vi "GEA2 Message to LEUI_LED with Binary conversion.vi"(5 "Ignore Brightness":bool, 7 "Raw Data In":string) -> (4 "Cycle Number":u32, 8 "LEUI_LEDs":T1)   [LabVIEW 2016, in "TLMB.lvlib"]
uses:
  Projects/TLMB.lvlib
  controls/LEUI_LEDs.ctl
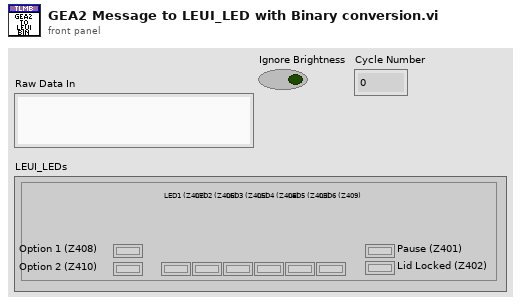
[diagram p1: front panel]
types:
  T1 = typedef "TLMB.lvlib/LEUI_LEDs.ctl" = cluster{"Pause (Z401)":bool, "Lid Locked (Z402)":bool, "LED1 (Z407)":bool, "LED2 (Z406)":bool, "LED3 (Z405)":bool, "LED4 (Z404)":bool, "LED5 (Z403)":bool, "LED6 (Z409)":bool, "Option 1 (Z408)":bool, "Option 2 (Z410)":bool}
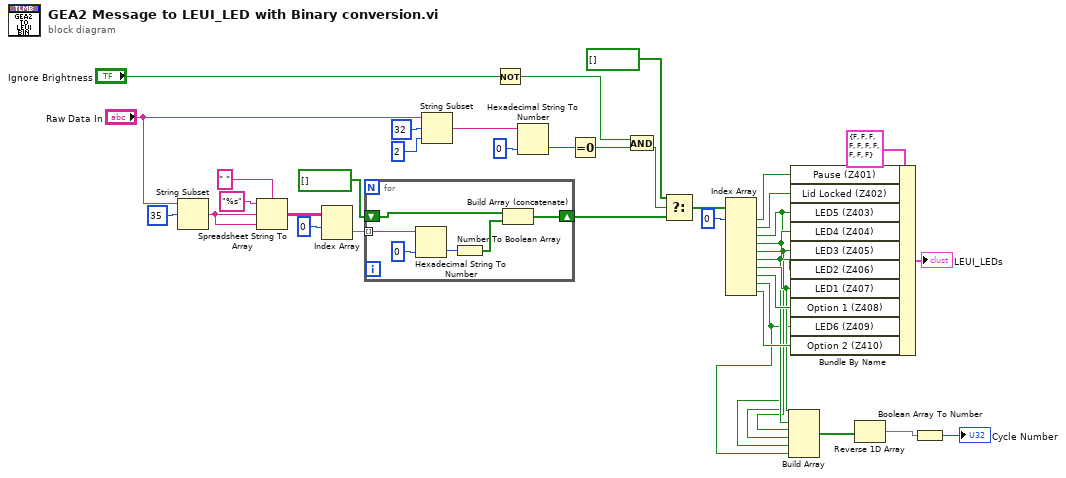
[diagram p0: block diagram]
diagram:
  n1 = String Subset(string="Raw Data In", offset (0)=35) -> (substring=w30:string)  [unwired: 1 in]
  n2 = Spreadsheet String To Array(delimiter (Tab)=" ", format string="%s", spreadsheet string=w30, array type (2D Dbl)=w30) -> (array=w34:string[][])
  n3 = Index Array(array=w34, index (row)=0) -> (element=w31:string[])  [unwired: 1 in]
  n4 = for {
    tunnel: w31 -> [w43] mode=indexing
    shift-right: [w39] -> w23
    shift-left: bool[] [] -> [w41]
    n5 = Hexadecimal String To Number(string=w43, default (0uL)=u8 0) -> (number=w42:u8)  [unwired: 1 in, 1 out]
    n6 = Number To Boolean Array(number=w42) -> (Boolean array=w40:bool[])
    n7 = Build Array (concatenate)(w41, w40) -> (w39:bool[])
  }
  n8 = String Subset(string="Raw Data In", offset (0)=32, length (rest)=2 ("length (rest)")) -> (substring=w27:string)
  n9 = Not(x="Ignore Brightness") -> (.not. x?=w10:bool)
  n10 = Hexadecimal String To Number(string=w27, default (0uL)=u32 0 ("default (0 U32)")) -> (number=w25:u32)  [unwired: 1 in, 1 out]
  n11 = Equal To 0?(x=w25) -> (x = 0?=w24:bool)
  n12 = And(x=w10, y=w24) -> (x .and. y?=w12:bool)
  n13 = Select(t=bool[] [], s=w12, f=w23) -> (s? t:f=w21:bool[])
  n14 = Index Array(array=w21, index #1=0 ("index")) -> (element #1=w20:bool, element #2=w17:bool, element #3=w5:bool, element #4=w6:bool, element #5=w7:bool, element #6=w8:bool, element #7=w9:bool, element #8=w14:bool, element #9=w4:bool, element #10=w13:bool)  [unwired: 9 in]
  n15 = Build Array(w9, w8, w7, w6, w5, w4) -> (w3:bool[])
  n16 = Bundle By Name(cluster=T1 {"Pause (Z401)"=FALSE, "Lid Locked (Z402)"=FALSE, "LED1 (Z407)"=FALSE, "LED2 (Z406)"=FALSE, "LED3 (Z405)"=FALSE, "LED4 (Z404)"=FALSE, "LED5 (Z403)"=FALSE, "LED6 (Z409)"=FALSE, "Option 1 (Z408)"=FALSE, "Option 2 (Z410)"=FALSE} ("LEUI_LEDs"), "Pause (Z401)"=w20, "Lid Locked (Z402)"=w17, "LED5 (Z403)"=w5, "LED4 (Z404)"=w6, "LED3 (Z405)"=w7, "LED2 (Z406)"=w8, "LED1 (Z407)"=w9, "Option 1 (Z408)"=w14, "LED6 (Z409)"=w4, "Option 2 (Z410)"=w13) -> (→"LEUI_LEDs":T1)
  n17 = Reverse 1D Array(array=w3) -> (reversed array=w2:bool[])
  n18 = Boolean Array To Number(Boolean array=w2) -> (number=→"Cycle Number":u32)
